vi "WavaFrequencyMeasurement3.vi"() -> ()   [LabVIEW 2019]
uses:
  <vilib>/Platform/TimedLoop/XDataNode/timing_clust.ctl
  <vilib>/Platform/TimedLoop/XDataNode/nitl_modes.ctl
  <vilib>/Platform/TimedLoop/XDataNode/wakeup.ctl
  <vilib>/rvi/Emulation/niFpgaSctlEmulationGetInTimedLoop.vi
  <vilib>/rvi/Emulation/niFpgaEmulationReportErrorSimple.vi
  <vilib>/rvi/Emulation/niFpgaGetClockAttributes.vi
  <vilib>/rvi/Emulation/niFpgaCriticalErrorInLSC.vi
  <vilib>/rvi/eio/common/nirviEmuTemplateMethod_errors.vi
  <vilib>/Platform/TimedLoop/XDataNode/XDataNode.xnode
  <vilib>/eio/EIONode/EIONode.xnode
  <vilib>/Platform/TimedLoop/XDataNode/XDNodeRunTimeDep.lvlib
panel:
  out "波形图表 2":cluster{u64, u64}(graph)
  out "时钟信号个数 2":u64
  out "被测信号个数 2":u64
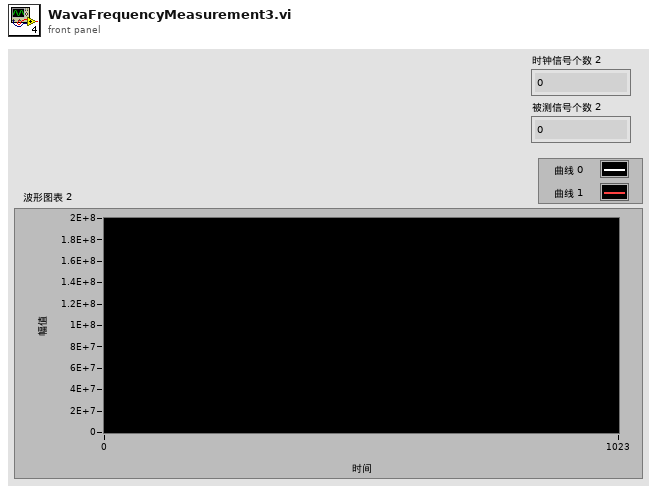
[diagram p1: front panel]
types:
  T1 = typedef "XDNodeRunTimeDep.lvlib/timing_clust.ctl" = cluster{"Expected End [f-1]":u64, "Actual End [f-1]":u64, "Finished Late? [f-1]":bool, "Expected End [i-1]":u64, "Actual End [i-1]":u64, "Finished Late? [i-1]":bool, "Expected Start [i]":u64, "Actual Start [i]":u64, "Expected Start [f]":u64, "Actual Start [f]":u64, "Source Name":string, "Structure Name":string, "Period":i64, "Deadline":i64, "Offset":i64, "Start":i64, "Priority":i32, "Timeout":i32, "Mode":T2, "Wakeup Reason":T3, "Error":errorcluster, "Source Type":string, "Secondary Source Type":string, "Global End Time":u64, "Global Start Time":u64, "Frame Duration":u64, "Iteration Duration":u64, "Assigned CPU":i32, "I/O Scan Engine Mode":u32}
  T2 = typedef "XDNodeRunTimeDep.lvlib/nitl_modes.ctl" = enum32{"No Change", "Process missed periods, maintain original phase", "Discard missed periods, maintain original phase", "Process missed periods, ignore original phase", "Discard missed periods, ignore original phase"}
  T3 = typedef "XDNodeRunTimeDep.lvlib/wakeup.ctl" = enum32{"Normal", "Aborted", "Asynchronous wakeup", "Timing source error", "Timed loop error", "Timeout"}
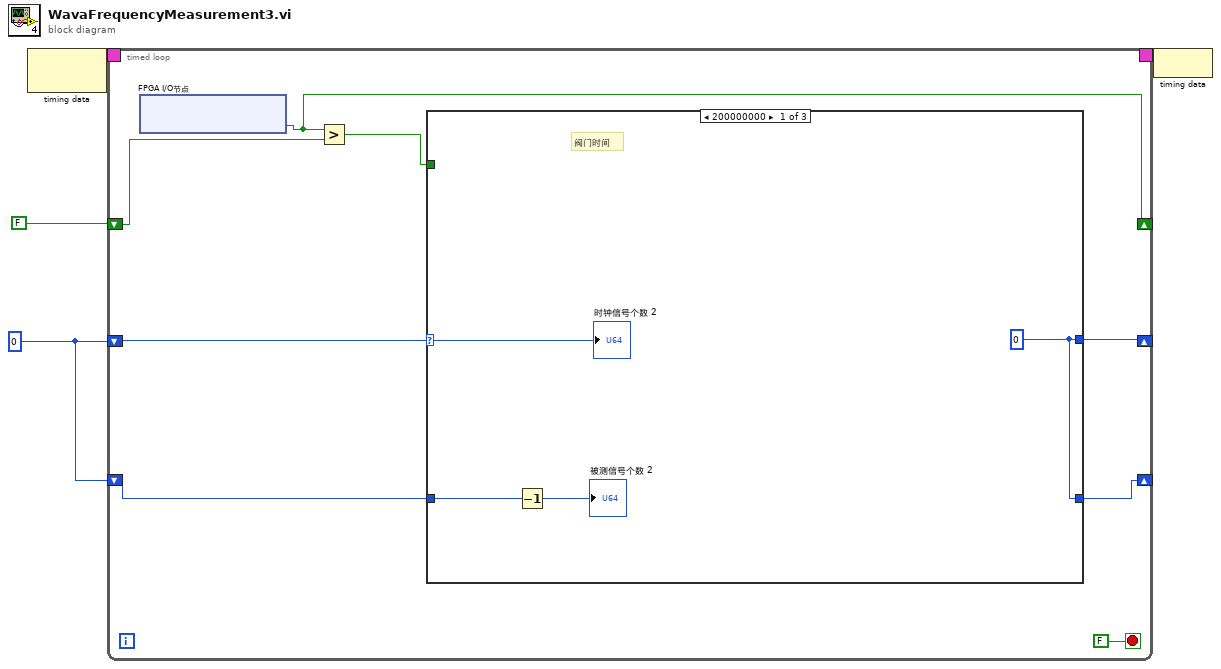
[diagram p0: block diagram]
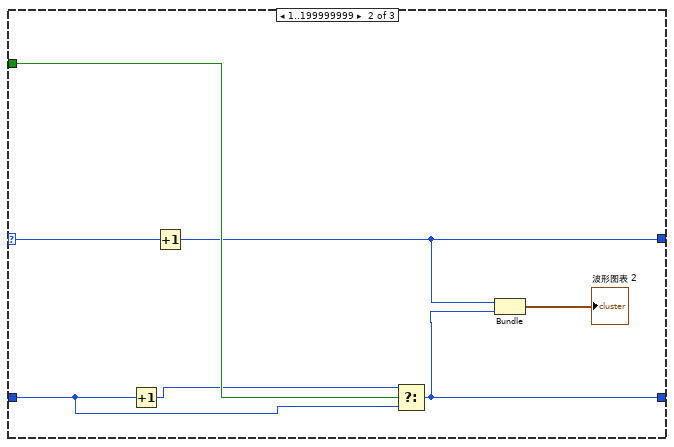
[diagram p2: hidden frame]
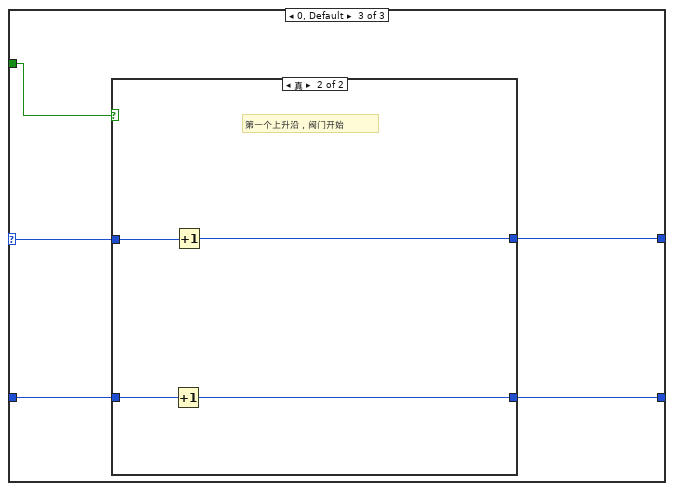
[diagram p3: hidden frame]
diagram:
  w2 = u64 0
  n1 = node-c288() -> (w4:T1)  [unwired: 1 in]
  n2 = timed-loop {
    timing: w4 -> [_]
    timing-out: [_] -> w3
    shift-right: [w11] -> _
    shift-left: FALSE -> [w12]
    shift-right: [w6] -> _
    shift-left: w2 -> [w9]
    shift-right: [w5] -> _
    shift-left: w2 -> [w8]
    stop <- FALSE stop-if-true
    n3 = xnode "FPGA I/O节点"() -> ("ConnectorB/DIO0"=w11:bool)  [unwired: 1 in, 1 out]
    n4 = Greater?(x=w11, y=w12) -> (0:w10:bool)
    n5 = case "条件结构" shown="200000000" w9 {
      selector: w9 -> [w15 w23 w27]
      tunnel: w10 -> [_ w21 w28]
      tunnel: w8 -> [w14 w22 w26]
      tunnel: [w16 w20 w25] -> w6
      tunnel: [w16 w18 w24] -> w5
      frame 200000000 {
        w16 = u64 0
        # "阀门时间"
        n6 = Decrement(x=w14) -> (x-1=→"被测信号个数 2":u64)
        "时钟信号个数 2" <- w15
      }
      frame 1..199999999 {
        n7 = Increment(x=w22) -> (x+1=w19:u64)
        n8 = Increment(x=w23) -> (x+1=w20:u64)
        n9 = Select(t=w19, s=w21, f=w22) -> (s? t:f=w18:u64)
        n10 = Bundle(w20, w18) -> (→"波形图表 2":cluster{u64, u64})  [unwired: 1 in]
      }
      frame 0, Default {
        n11 = case shown="真" w28 {
          tunnel: w27 -> [w30 w34]
          tunnel: w26 -> [w29 w33]
          tunnel: [w30 w32] -> w25
          tunnel: [w29 w31] -> w24
          frame False {
            # "不开始"
          }
          frame True {
            # "第一个上升沿，阀门开始"
            n12 = Increment(x=w33) -> (x+1=w31:u64)
            n13 = Increment(x=w34) -> (x+1=w32:u64)
          }
        }
      }
    }
  }
  n14 = node-c288(w3) -> ()
